vi "FdxCmdTMGetTSListCvi.vi"(8 "error in":errorcluster, 10 "TMHandle":u32, 11 "InstrumentHandle":u32) -> (0 "error out":errorcluster, 1 "GetTSList":T1, 2 "TMHandleOut":u32, 3 "InstrumentHandle":u32)   [LabVIEW 2020, in "AIM664LV.lvlib"]
doc: "This function is used to get the current Time Manager TS_List. This function can be called while a Time Manager is running."
uses:
  AIM664LV.lvlib
  AFDX_LibraryAdmin/FdxGlobalDllPath.vi
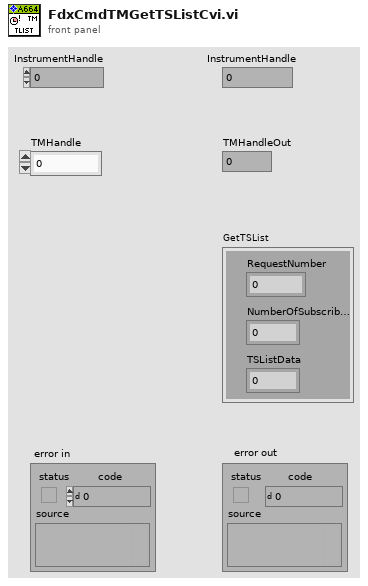
[diagram p1: front panel]
types:
  T1 = cluster{"RequestNumber":u16, "NumberOfSubscribers":u16, "TSListData":u32}
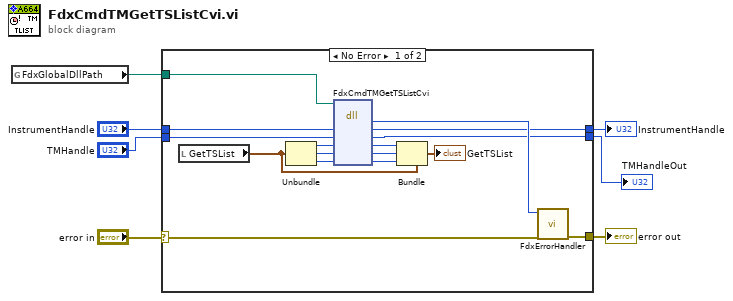
[diagram p0: block diagram]
diagram:
  n1 = global read "FdxGlobalDllPath.vi" "FdxGlobalDllPath"() -> (w5:path)
  n2 = case shown="No Error" "error in" {
    selector: "error in" -> [w22 w26]
    tunnel: [w23 w26] -> w7
    tunnel: w5 -> [w13 _]
    tunnel: "InstrumentHandle" -> [w12 w25]
    tunnel: [w11 w25] -> w3
    tunnel: "TMHandle" -> [w10 w24]
    tunnel: [w8 w24] -> w1
    frame No Error {
      n3 = local read "GetTSList"() -> (w9:T1)
      n4 = Unbundle(w9) -> ("RequestNumber"=w16:u16, "NumberOfSubscribers"=w15:u16, "TSListData"=w14:u32)
      n5 = dll-call lib="aim_fdx.19.dll" fn="FdxCmdTMGetTSListCvi"(path in=w13, "InstrumentHandle"=w12, "TMHandle"=w10, "RequestNumber"=w16, "NumberofSubscribers"=w15, "TSListData"=w14) -> ("status"=w21:i32, "InstrumentHandle"=w11:u32, "TMHandle"=w8:u32, "RequestNumber"=w20:u16, "NumberofSubscribers"=w19:u16, "TSListData"=w18:u32)  [unwired: 2 in, 2 out]
      n6 = Bundle(cluster=w9, "RequestNumber"=w20, "NumberOfSubscribers"=w19, "TSListData"=w18) -> (→"GetTSList":T1)
      n7 = call "FdxErrorHandler.vi"("error in"=w22, "AIM Error"=w21) -> ("error out"=w23:errorcluster)  [unwired: 9 in]
    }
    frame Error {
    }
  }
  "error out" <- w7
  "InstrumentHandle" <- w3
  "TMHandleOut" <- w1
